vi "multi-graph-example.vi"() -> ()   [LabVIEW 2017]
panel:
  out "cycle #":i32
  in  "LSI-U CH labels":string[](array[string])
  out "labels S1":string[](array[string])
  in  "GraphU2 SEL":i32[](array[numeric])
  in  "log/linear":bool
  in  "stop":bool
  out "Graph1 (4-10K)":cluster{timestamp[], dbl[]}[](graph)
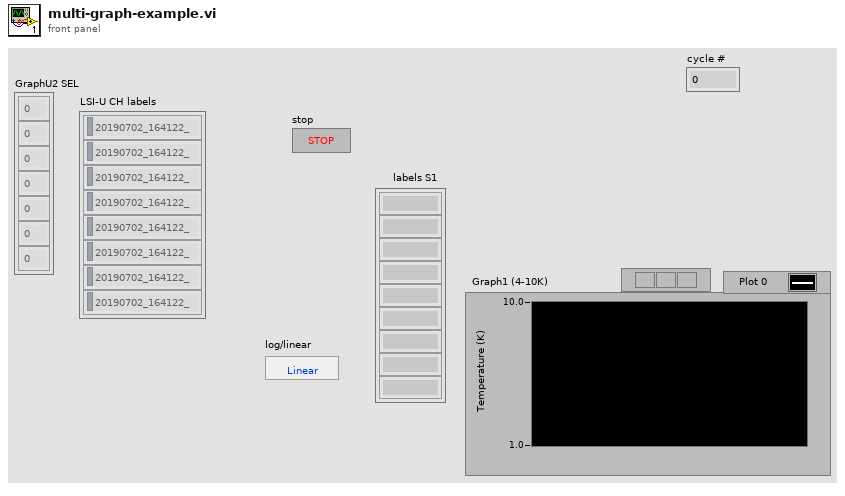
[diagram p1: front panel]
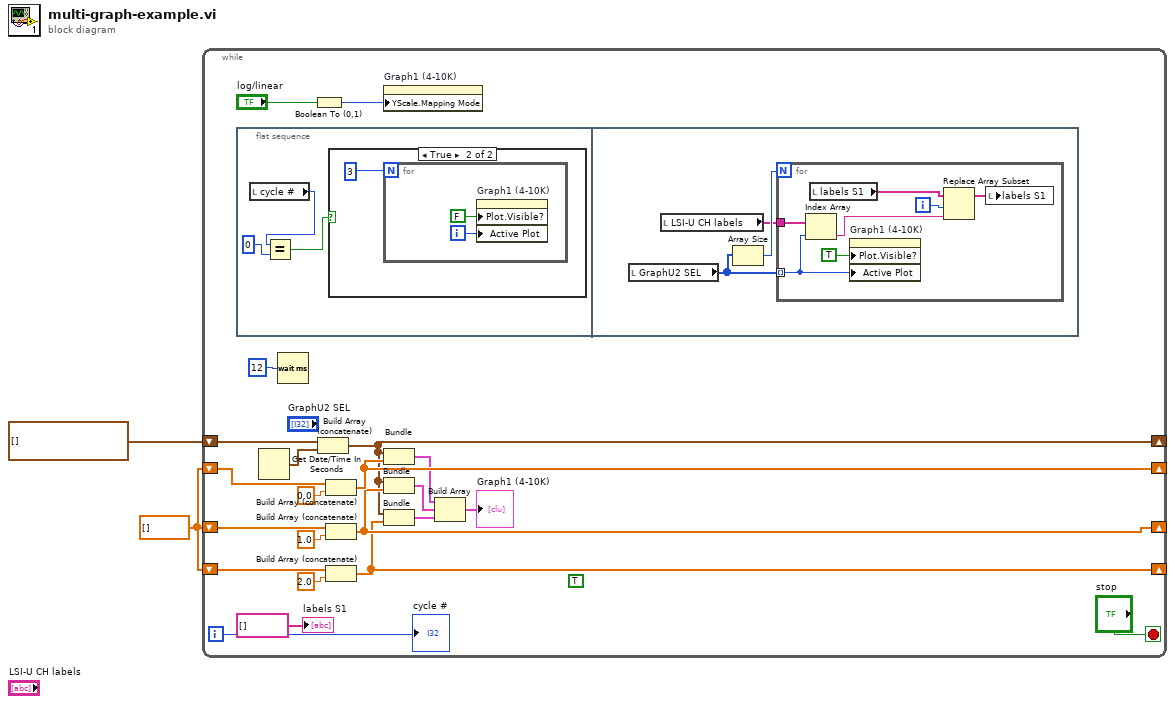
[diagram p0: block diagram]
diagram:
  w1 = dbl[] []
  n1 = while {
    shift-right: [w18] -> _
    shift-left: w1 -> [w23]
    shift-right: [w12] -> _
    shift-left: timestamp[] [] -> [w21]
    shift-right: [w15] -> _
    shift-left: w1 -> [w16]
    shift-right: [w11] -> _
    shift-left: w1 -> [w13]
    i -> [w3]
    stop <- "stop" stop-if-true
    (unwired) TRUE ("Visible")
    n2 = flat-sequence {
      frame #0 {
        n3 = local read "cycle #"() -> (w27:i32)
        n4 = Equal?(x=w27, y=0 ("x")) -> (x = y?=w25:bool)
        n5 = case shown="True" w25 {
          frame False {
          }
          frame True {
            n6 = for {
              N: 3 -> [_]
              i -> [w30]
              n7 = property on="Graph1 (4-10K)" class="XYGraph (strict)"("Plot.Visible?"=FALSE ("Plot.Visible"), "Active Plot"=w30) -> ()  [unwired: 2 in, 2 out]
            }
          }
        }
      }
      frame #1 {
        n8 = local read "GraphU2 SEL"() -> (w32:i32[])
        n9 = local read "LSI-U CH labels"() -> (w31:string[])
        n10 = Array Size(array=w32) -> (size(s)=w33:i32)
        n11 = for {
          N: w33 -> [_]
          tunnel: w32 -> [w38] mode=indexing
          tunnel: w31 -> [w39]
          i -> [w36]
          n12 = Index Array(array=w39, index=w38) -> (element=w35:string)
          n13 = local read "labels S1"() -> (w37:string[])
          n14 = property on="Graph1 (4-10K)" class="XYGraph (strict)"("Plot.Visible?"=TRUE ("Plot.Visible"), "Active Plot"=w38) -> ()  [unwired: 2 in, 2 out]
          n15 = Replace Array Subset(array=w37, new element=w35, index=w36) -> (w34:string[])
          n16 = local write "labels S1"(w34) -> ()
        }
      }
    }
    n17 = Get Date/Time In Seconds() -> (seconds since 1Jan1904=w22:timestamp)
    n18 = Wait (ms)(milliseconds to wait=u32 12) -> ()  [unwired: 1 out]
    n19 = Boolean To (0,1)(Boolean="log/linear") -> (0, 1=w5:i16)
    n20 = Build Array (concatenate)(w21, w22) -> (w12:timestamp[])
    n21 = Build Array (concatenate)(w23, 0.0) -> (w18:dbl[])
    n22 = Build Array (concatenate)(w16, 1.0) -> (w15:dbl[])
    n23 = Build Array (concatenate)(w13, 2.0) -> (w11:dbl[])
    n24 = property on="Graph1 (4-10K)" class="XYGraph (strict)"("YScale.Mapping Mode"=w5) -> ()  [unwired: 2 in, 2 out]
    n25 = Bundle(w12, w18) -> (w10:cluster{timestamp[], dbl[]})  [unwired: 1 in]
    n26 = Bundle(w12, w15) -> (w9:cluster{timestamp[], dbl[]})  [unwired: 1 in]
    n27 = Bundle(w12, w11) -> (w8:cluster{timestamp[], dbl[]})  [unwired: 1 in]
    n28 = Build Array(w10, w9, w8) -> (→"Graph1 (4-10K)":cluster{timestamp[], dbl[]}[])
    "labels S1" <- string[] []
    "cycle #" <- w3
  }
